vi "Consumer.vi"(8 "error in (no error)":errorcluster, 9 "Data":variant, 10 "Case ID":string, 11 "uService Template in":refnum<class "Detector Manager.lvclass">) -> (0 "error out":errorcluster, 3 "uService Template out":refnum<class "Detector Manager.lvclass">)   [LabVIEW 2026, in "TALOS.lvlib" / "Detector Manager.lvlib" / "Detector Manager.lvclass"]
uses:
  Detector Manager.lvclass
  C:/LabVIEW Code/TALOS/talos/Father of all uServices/Father of all uServices/Father of all uServices.lvclass
  Detector Manager Consumer Case Selector.ctl
  Detector Manager.lvclass/Detector Manager.ctl
  Ancestor/Ancestor/Ancestor.lvclass/Ancestor.ctl
  Father of all uServices/Father of all uServices/Father of all uServices.lvclass/Father of all uServices.ctl
  Father of all uServices/Father of all uServices Messages/Consumer Msg/Consumer Msg.lvclass/Consumer Msg.ctl
  Support VIs/Generate Error.vi
  FGV/Error Memory/Get Error Description.vi
  Support VIs/Get PC name.vi
  Ancestor/Ancestor/Read ID.vi
  Support VIs/Get Class Name.vi
  FGV/Error Memory/Error Memory Core.vi
  <vilib>/AdvancedString/Delimited String to 1D String Array.vi
  <vilib>/AdvancedString/Delimited String to 1D String Array (string).vi
  Support VIs/Circus Root Path.vi
  FGV/Error Memory/Error Crt Lvl checker.vi
  FGV/Error Memory/Error Memory Core.vi/40c8088d-b597-4017-91af-faa98e00292e.vi
  FGV/Error Memory/Error Memory Core.vi/d4a3ab98-063c-4e44-b43d-fbdcfe6c2be2.vi
  Father of all uServices/Father of all uServices/Father of all uServices.lvclass
  C:/LabVIEW Code/TALOS/builds/Actor Framework PPL/Actor Framework.lvlibp/1abvi3w/vi.lib/ActorFramework/Actor/Actor.lvclass
  Support VIs/Global Memory.vi
  <vilib>/Utility/LVClass/Get LV Class Name.vi
  Support VIs/Is in Packed Library.vi
  Support VIs/TALOS Root path.vi
  Support VIs/Read CSV worksheet.vi
  Support VIs/Global Constants.vi
  <vilib>/Utility/error.llb/General Error Handler.vi
  Support VIs/Error Log.vi
  builds/Actor Framework PPL/Actor Framework.lvlibp/1abvi3w/vi.lib/ActorFramework/Actor/Read Self Enqueuer.vi
  <userlib>/_OpenG.lib/lvdata/lvdata.llb/Get Strings from Enum__ogtk.vi
  builds/Actor Framework PPL/Actor Framework.lvlibp/1abvi3w/vi.lib/ActorFramework/Message Enqueuer/Enqueue.vi
  Ancestor/Ancestor/Ancestor.lvclass
  <vilib>/Comparison/Equal/Equal Functor/Equal Functor.lvclass
  Father of all uServices/Father of all uServices Messages/Consumer Msg/Consumer Msg.lvclass
  Classes/Father of all Detectors/Father Of All Detectors.lvclass
  TALOS.lvlib
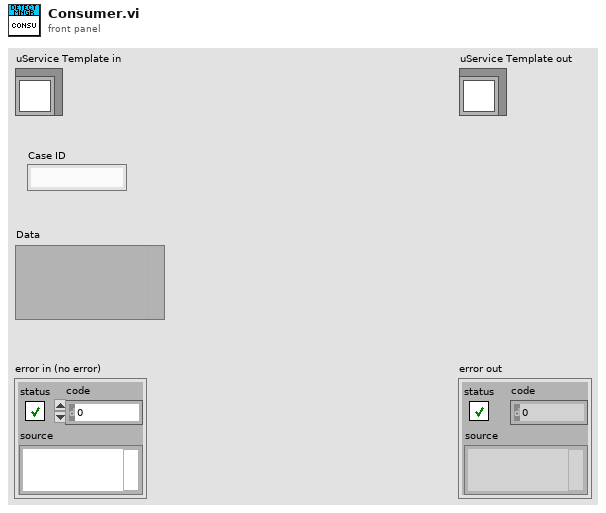
[diagram p1: front panel]
types:
  T1 = typedef "TALOS.lvlib/Detector Manager.lvlib/Detector Manager.lvclass/Detector Manager Consumer Case Selector.ctl" = enum16{"Set Configuration", "Arm", "Acquiring", "Save Data", "Self Check", "Safe Mode", "Init", "Close", "Stop"}
  T2 = typedef "TALOS.lvlib/Father Of All Detectors.lvlib/Father Of All Detectors.lvclass/Detector Settings.ctl" = cluster{"Stop after Save Data?":bool, "Stop before ReArm?":bool}
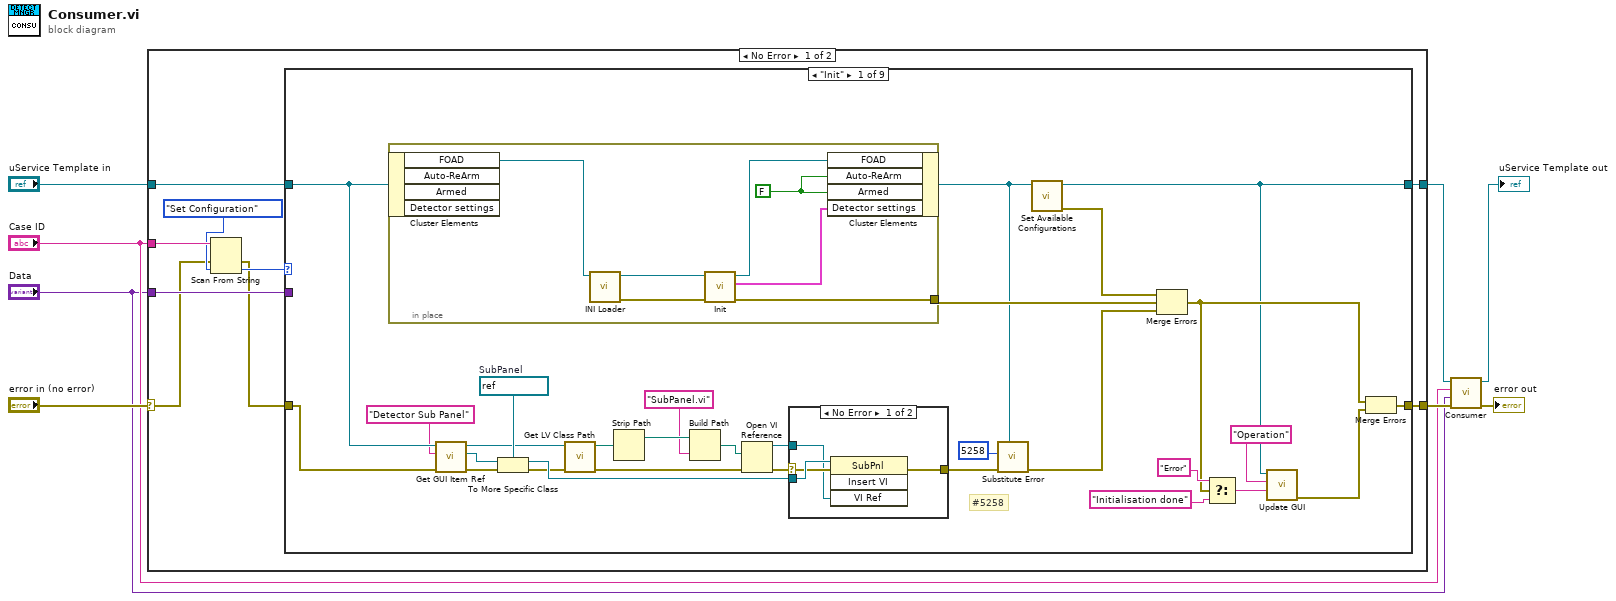
[diagram p0: block diagram]
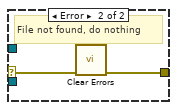
[diagram p2: hidden frame]
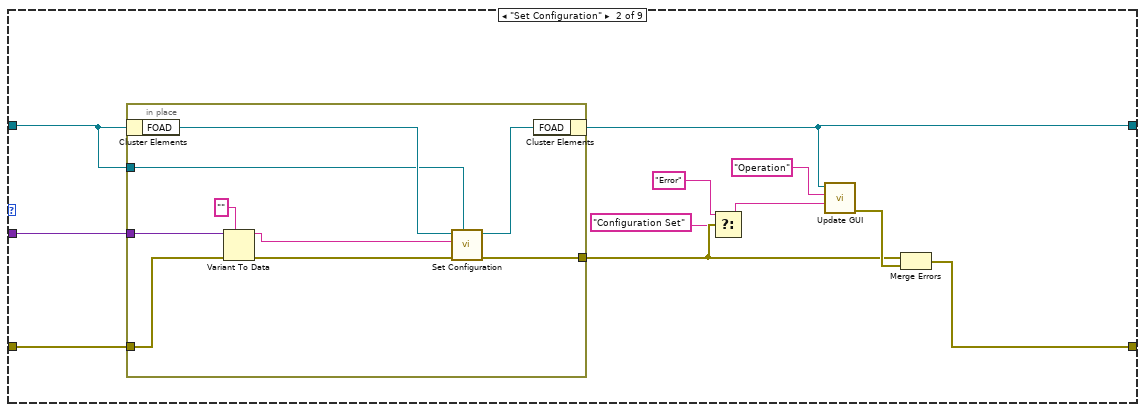
[diagram p3: hidden frame]
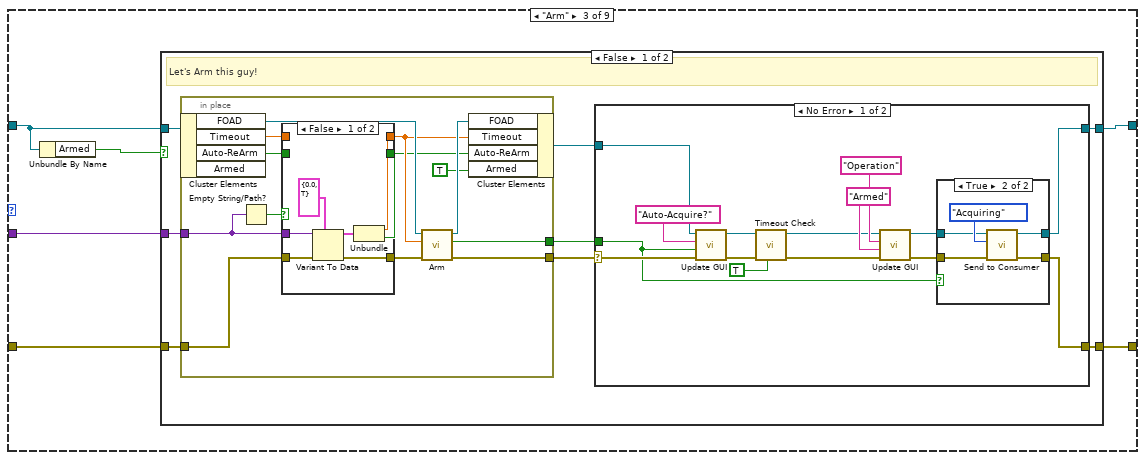
[diagram p4: hidden frame]
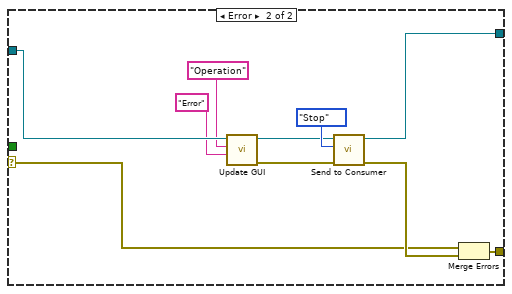
[diagram p7: hidden frame]
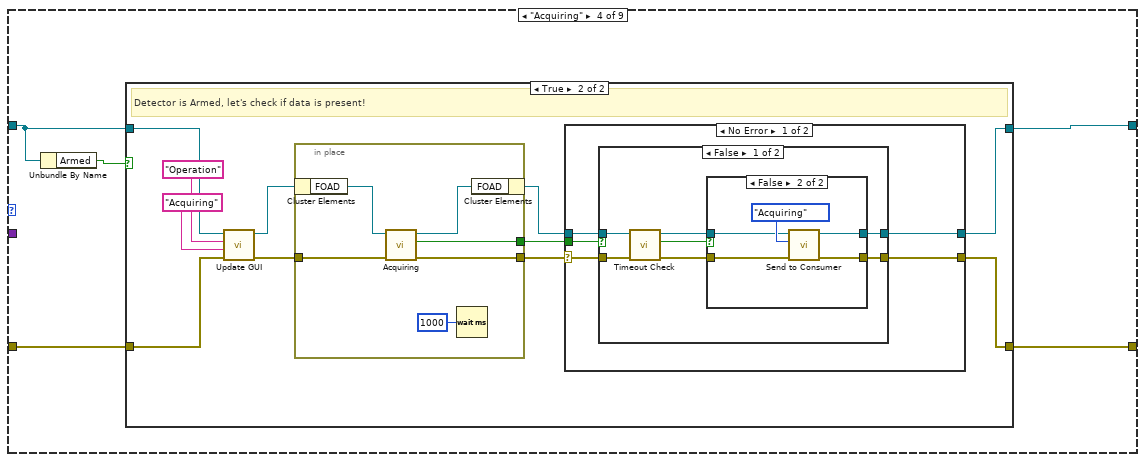
[diagram p9: hidden frame]
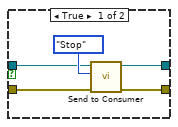
[diagram p11: hidden frame]
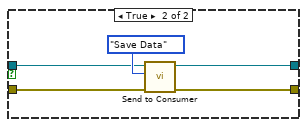
[diagram p12: hidden frame]
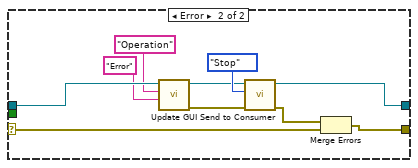
[diagram p13: hidden frame]
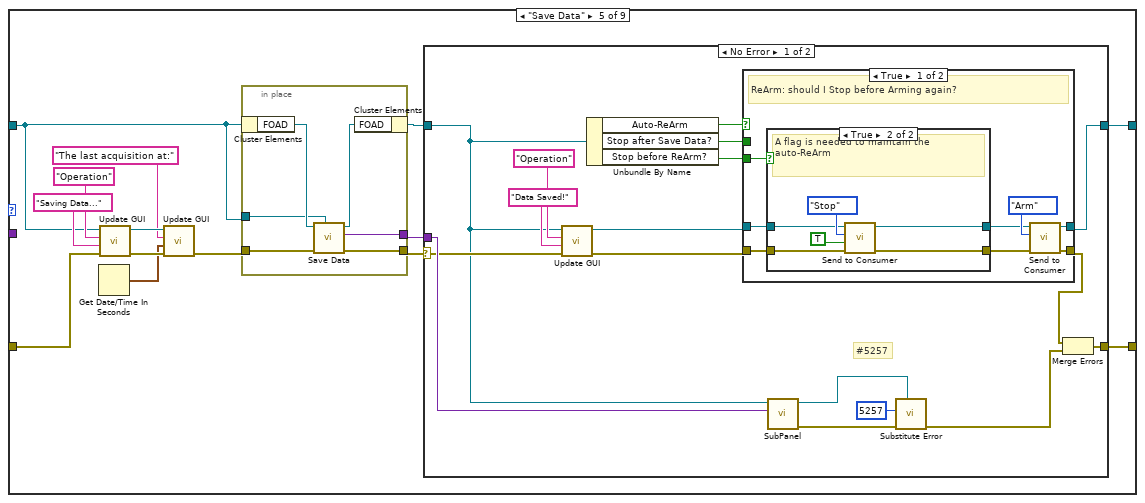
[diagram p14: hidden frame]
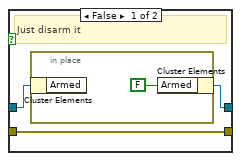
[diagram p15: hidden frame]
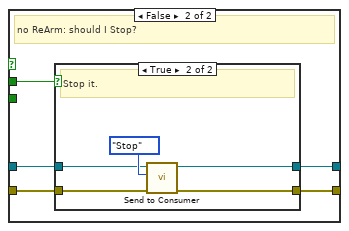
[diagram p16: hidden frame]
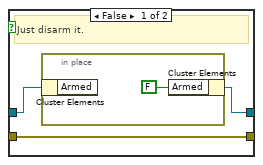
[diagram p17: hidden frame]
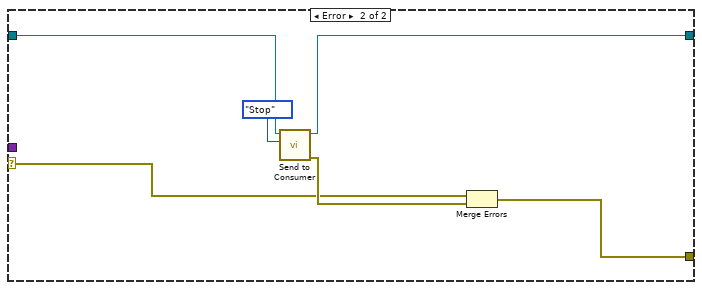
[diagram p18: hidden frame]
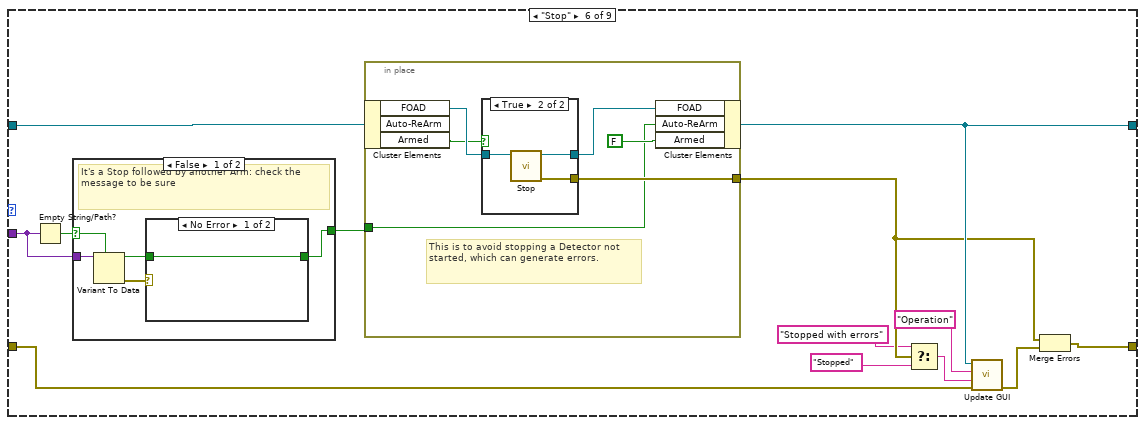
[diagram p19: hidden frame]
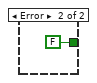
[diagram p20: hidden frame]
diagram:
  n1 = case shown="No Error" "error in (no error)" {
    selector: "error in (no error)" -> [w10 w392]
    tunnel: "uService Template in" -> [w16 w393]
    tunnel: [w14 w393] -> w4
    tunnel: [w15 w392] -> w3
    tunnel: "Case ID" -> [w13 _]
    tunnel: "Data" -> [w17 _]
    frame No Error {
      n2 = Scan From String(input string=w13, error in=w10, default 1=Detector_Manager_Consumer_Case_Selector."Set Configuration") -> (error out=w9:errorcluster, output 1=w11:T1)  [unwired: 2 in, 2 out]
      n3 = case shown="\"Init\"" w11 {
        tunnel: w17 -> [_ w71 w86 _ _ w289 _ w336 w375]
        tunnel: w9 -> [w39 w70 w85 w154 w224 w295 w327 w349 w373]
        tunnel: w16 -> [w40 w61 w82 w153 w218 w300 w328 w350 w374]
        tunnel: [w44 w65 w83 w155 w221 w296 w320 w341 w367] -> w15
        tunnel: [w19 w67 w84 w156 w223 w297 w324 w338 w364] -> w14
        frame "Init" {
          w35 = refnum<vi> refnum  # SubPanel
          # "#5258"
          n4 = in-place "In Place Element Structure" {
            in-place-border: [w59] -> w43
            w58 = FALSE ("Armed")
            n5 = in-place-cluster #1(w40) -> ("FOAD"=w56:refnum<class "Father Of All Detectors.lvclass">)  [unwired: 3 out]
            n6 = call-dynamic "INI Loader.vi"("Father Of All Detectors in"=w56) -> ("error out"=w54:errorcluster, "Father Of All Detectors out"=w55:refnum<class "Father Of All Detectors.lvclass">)  [unwired: 9 in]
            n7 = call-dynamic "Init.vi"("error in (no error)"=w54, "Father Of All Detectors in"=w55) -> ("error out"=w59:errorcluster, "Detector Settings"=w57:T2, "Father Of All Detectors out"=w60:refnum<class "Father Of All Detectors.lvclass">)  [unwired: 7 in]
            n8 = in-place-cluster #1("FOAD"=w60, "Auto-ReArm"=w58, "Armed"=w58, "Detector settings"=w57) -> (w20:refnum<class "Detector Manager.lvclass">)
          }
          n9 = call "Get GUI Item Ref.vi"("error in (no error)"=w39, "FP Item Name"="Detector Sub Panel", "uService Template in"=w40) -> ("error out"=w36:errorcluster, "Ctl Refnum"=w37:refnum<vi>, "uService Template out"=w33:refnum<class "Detector Manager.lvclass">)  [unwired: 6 in]
          n10 = To More Specific Class(target class=w35, reference=w37, error in=w36) -> (specific class reference=w34:refnum<vi>, error out=w32:errorcluster)
          n11 = call <vilib>:"Get LV Class Path.vi"("error in (no error)"=w32, "object"=w33) -> ("error out"=w28:errorcluster, "class path"=w31:path)  [unwired: 8 in]
          n12 = Strip Path(path=w31) -> (stripped path=w30:path)  [unwired: 1 out]
          n13 = Build Path(base path=w30, name or relative path="SubPanel.vi") -> (appended path=w27:path)
          n14 = Open VI Reference(vi path=w27, error in (no error)=w28) -> (vi reference=w25:refnum<vi>, error out=w26:errorcluster)  [unwired: 4 in]
          n15 = case shown="No Error" w26 {
            selector: w26 -> [w50 w53]
            tunnel: w34 -> [w51 _]
            tunnel: w25 -> [w49 _]
            tunnel: [w48 w52] -> w23
            frame No Error {
              n16 = invoke class="SubPnl" method="Insert VI"(reference=w51, error in=w50, "VI Ref"=w49) -> (error out=w48:errorcluster)  [unwired: 1 in, 3 out]
            }
            frame Error {
              # "File not found, do nothing"
              n17 = call <vilib>:"Clear Errors.vi"("error in (no error)"=w53) -> ("error out"=w52:errorcluster)  [unwired: 5 in, 1 out]
            }
          }
          n18 = call "Substitute Error.vi"("LabVIEW Object"=w20, "error in (no error)"=w23, "Error Code"=5258) -> ("error out"=w22:errorcluster)  [unwired: 8 in]
          n19 = call "Set Available Configurations.vi"("Detector Manager in"=w20) -> ("error out"=w18:errorcluster, "Detector Manager out"=w19:refnum<class "Detector Manager.lvclass">)  [unwired: 9 in]
          n20 = Merge Errors(w18, w43, w22) -> (w24:errorcluster)
          n21 = Select(t="Error" ("GUI Item Name"), s=w24, f="Initialisation done" ("GUI Item Name")) -> (s? t:f=w45:string)
          n22 = call "Update GUI.vi"("Data"=w45, "GUI Item Name"="Operation", "uService Template in"=w19) -> ("error out"=w46:errorcluster)  [unwired: 7 in, 1 out]
          n23 = Merge Errors(w24, w46) -> (w44:errorcluster)
        }
        frame "Set Configuration" {
          n24 = in-place "In Place Element Structure" {
            in-place-border: w71 -> [w74]
            in-place-border: w70 -> [w80]
            in-place-border: [w76] -> w64
            in-place-border: w61 -> [w72]
            n25 = in-place-cluster #2(w61) -> ("FOAD"=w79:refnum<class "Father Of All Detectors.lvclass">)
            n26 = Variant To Data(error in=w80, type="", Variant=w74) -> (data=w77:string, error out=w75:errorcluster)
            n27 = call-dynamic "Set Configuration.vi"("Detector Manager"=w72, "error in (no error)"=w75, "Configuration Name"=w77, "Father Of All Detectors in"=w79) -> ("error out"=w76:errorcluster, "Father Of All Detectors out"=w78:refnum<class "Father Of All Detectors.lvclass">)  [unwired: 6 in]
            n28 = in-place-cluster #2("FOAD"=w78) -> (w67:refnum<class "Detector Manager.lvclass">)
          }
          n29 = Select(t="Error" ("f"), s=w64, f="Configuration Set" ("GUI Item Name")) -> (s? t:f=w66:string)
          n30 = call "Update GUI.vi"("Data"=w66, "GUI Item Name"="Operation", "uService Template in"=w67) -> ("error out"=w68:errorcluster)  [unwired: 7 in, 1 out]
          n31 = Merge Errors(w64, w68) -> (w65:errorcluster)
        }
        frame "Arm" {
          n32 = Unbundle By Name(w82) -> ("Armed"=w81:bool)
          n33 = case shown="False" w81 {
            tunnel: w86 -> [w94 _]
            tunnel: w82 -> [w93 w151]
            tunnel: w85 -> [w92 w150]
            tunnel: [w88 w151] -> w84
            tunnel: [w87 w150] -> w83
            frame False {
              # "Let's Arm this guy!"
              n34 = in-place "In Place Element Structure" {
                in-place-border: w94 -> [w101]
                in-place-border: w92 -> [w104]
                in-place-border: [w103] -> w91
                in-place-border: [w102] -> w90
                n35 = in-place-cluster #3(w93) -> ("FOAD"=w107:refnum<class "Father Of All Detectors.lvclass">, "Timeout"=w99:dbl, "Auto-ReArm"=w97:bool)  [unwired: 1 out]
                n36 = Empty String/Path?(string/path=w101) -> (empty?=w100:bool)
                n37 = case shown="False" w100 {
                  tunnel: [w109 w116] -> w98
                  tunnel: [w113 w117] -> w105
                  tunnel: w104 -> [w112 w117]
                  tunnel: w101 -> [w111 _]
                  tunnel: w99 -> [_ w116]
                  tunnel: w97 -> [_ w115]
                  tunnel: [w108 w115] -> w96
                  frame False {
                    n38 = Variant To Data(error in=w112, type=cluster{dbl, bool} {0.0, TRUE}, Variant=w111) -> (data=w114:cluster{dbl, bool}, error out=w113:errorcluster)
                    n39 = Unbundle(w114) -> (w109:dbl, w108:bool)
                  }
                  frame True {
                  }
                }
                n40 = call-dynamic "Arm.vi"("error in (no error)"=w105, "Timeout (s)"=w98, "Father Of All Detectors in"=w107) -> ("error out"=w103:errorcluster, "Acquire?"=w102:bool, "Father Of All Detectors out"=w106:refnum<class "Father Of All Detectors.lvclass">)  [unwired: 6 in]
                n41 = in-place-cluster #3("FOAD"=w106, "Timeout"=w98, "Auto-ReArm"=w96, "Armed"=TRUE) -> (w89:refnum<class "Detector Manager.lvclass">)
              }
              n42 = case shown="No Error" w91 {
                selector: w91 -> [w132 w141]
                tunnel: w90 -> [w130 _]
                tunnel: w89 -> [w129 w149]
                tunnel: [w128 w148] -> w88
                tunnel: [w127 w142] -> w87
                frame No Error {
                  n43 = call "Update GUI.vi"("error in (no error)"=w132, "Data"=w130, "GUI Item Name"="Auto-Acquire?", "uService Template in"=w129) -> ("error out"=w120:errorcluster, "uService Template out"=w122:refnum<class "Detector Manager.lvclass">)  [unwired: 6 in]
                  n44 = call-dynamic "Timeout Check.vi"("Start"=TRUE, "error in (no error)"=w120, "Detector Manager in"=w122) -> ("error out"=w119:errorcluster, "Detector Manager out"=w121:refnum<class "Detector Manager.lvclass">)  [unwired: 6 in, 1 out]
                  n45 = call "Update GUI.vi"("error in (no error)"=w119, "Data"="Armed" ("GUI Item Name"), "GUI Item Name"="Operation", "uService Template in"=w121) -> ("error out"=w125:errorcluster, "uService Template out"=w124:refnum<class "Detector Manager.lvclass">)  [unwired: 6 in]
                  n46 = case shown="True" w130 {
                    tunnel: w125 -> [w133 w138]
                    tunnel: w124 -> [w134 w135]
                    tunnel: [w134 w137] -> w128
                    tunnel: [w133 w136] -> w127
                    frame False {
                    }
                    frame True {
                      n47 = call "Send to Consumer.vi"("error in (no error)"=w138, "Case ID"=Detector_Manager_Consumer_Case_Selector."Acquiring", "uService Template in"=w135) -> ("error out"=w136:errorcluster, "uService Template out"=w137:refnum<class "Detector Manager.lvclass">)  [unwired: 7 in]
                    }
                  }
                }
                frame Error {
                  n48 = call "Update GUI.vi"("Data"="Error" ("GUI Item Name"), "GUI Item Name"="Operation", "uService Template in"=w149) -> ("error out"=w145:errorcluster, "uService Template out"=w140:refnum<class "Detector Manager.lvclass">)  [unwired: 7 in]
                  n49 = call "Send to Consumer.vi"("error in (no error)"=w145, "Case ID"=Detector_Manager_Consumer_Case_Selector."Stop", "uService Template in"=w140) -> ("error out"=w147:errorcluster, "uService Template out"=w148:refnum<class "Detector Manager.lvclass">)  [unwired: 7 in]
                  n50 = Merge Errors(w141, w147) -> (w142:errorcluster)
                }
              }
            }
            frame True {
              # "Armed pressed twice, ignore the second."
            }
          }
        }
        frame "Acquiring" {
          n51 = Unbundle By Name(w153) -> ("Armed"=w152:bool)
          n52 = case shown="True" w152 {
            tunnel: [w158 w169] -> w156
            tunnel: [w157 w168] -> w155
            tunnel: w154 -> [w157 w165]
            tunnel: w153 -> [w158 w159]
            frame False {
              # "This is a spurious message, just ignore it (it can happen if during an acquisition, the Stop button get pressed)."
            }
            frame True {
              # "Detector is Armed, let's check if data is present!"
              n53 = call "Update GUI.vi"("error in (no error)"=w165, "Data"="Acquiring" ("GUI Item Name"), "GUI Item Name"="Operation", "uService Template in"=w159) -> ("error out"=w163:errorcluster, "uService Template out"=w164:refnum<class "Detector Manager.lvclass">)  [unwired: 6 in]
              n54 = in-place "In Place Element Structure" {
                in-place-border: [w210] -> w160
                in-place-border: [w209] -> w162
                in-place-border: w163 -> [w207]
                n55 = in-place-cluster #4(w164) -> ("FOAD"=w212:refnum<class "Father Of All Detectors.lvclass">)
                n56 = call-dynamic "Acquiring.vi"("error in (no error)"=w207, "Father Of All Detectors in"=w212) -> ("error out"=w210:errorcluster, "Ready to Save Data?"=w209:bool, "Father Of All Detectors out"=w211:refnum<class "Father Of All Detectors.lvclass">)  [unwired: 7 in]
                n57 = Wait (ms)(milliseconds to wait=u32 1000) -> ()  [unwired: 1 out]
                n58 = in-place-cluster #4("FOAD"=w211) -> (w161:refnum<class "Detector Manager.lvclass">)
              }
              n59 = case shown="No Error" w160 {
                selector: w160 -> [w170 w200]
                tunnel: [w174 w201] -> w169
                tunnel: [w173 w199] -> w168
                tunnel: w162 -> [w172 _]
                tunnel: w161 -> [w171 w206]
                frame No Error {
                  n60 = case shown="False" w172 {
                    tunnel: [w181 w195] -> w174
                    tunnel: [w180 w194] -> w173
                    tunnel: w171 -> [w179 w192]
                    tunnel: w170 -> [w178 w193]
                    frame False {
                      n61 = call-dynamic "Timeout Check.vi"("error in (no error)"=w178, "Detector Manager in"=w179) -> ("error out"=w177:errorcluster, "Timeout"=w175:bool, "Detector Manager out"=w176:refnum<class "Detector Manager.lvclass">)  [unwired: 7 in]
                      n62 = case shown="False" w175 {
                        tunnel: [w185 w190] -> w181
                        tunnel: [w184 w189] -> w180
                        tunnel: w176 -> [w182 w187]
                        tunnel: w177 -> [w183 w188]
                        frame True {
                          n63 = call "Send to Consumer.vi"("error in (no error)"=w183, "Case ID"=Detector_Manager_Consumer_Case_Selector."Stop", "uService Template in"=w182) -> ("error out"=w184:errorcluster, "uService Template out"=w185:refnum<class "Detector Manager.lvclass">)  [unwired: 7 in]
                        }
                        frame False {
                          n64 = call "Send to Consumer.vi"("error in (no error)"=w188, "Case ID"=Detector_Manager_Consumer_Case_Selector."Acquiring", "uService Template in"=w187) -> ("error out"=w189:errorcluster, "uService Template out"=w190:refnum<class "Detector Manager.lvclass">)  [unwired: 7 in]
                        }
                      }
                    }
                    frame True {
                      n65 = call "Send to Consumer.vi"("error in (no error)"=w193, "Case ID"=Detector_Manager_Consumer_Case_Selector."Save Data", "uService Template in"=w192) -> ("error out"=w194:errorcluster, "uService Template out"=w195:refnum<class "Detector Manager.lvclass">)  [unwired: 7 in]
                    }
                  }
                }
                frame Error {
                  n66 = call "Update GUI.vi"("Data"="Error" ("GUI Item Name"), "GUI Item Name"="Operation", "uService Template in"=w206) -> ("error out"=w202:errorcluster, "uService Template out"=w197:refnum<class "Detector Manager.lvclass">)  [unwired: 7 in]
                  n67 = call "Send to Consumer.vi"("error in (no error)"=w202, "Case ID"=Detector_Manager_Consumer_Case_Selector."Stop", "uService Template in"=w197) -> ("error out"=w198:errorcluster, "uService Template out"=w201:refnum<class "Detector Manager.lvclass">)  [unwired: 7 in]
                  n68 = Merge Errors(w198, w200) -> (w199:errorcluster)
                }
              }
            }
          }
        }
        frame "Save Data" {
          n69 = Get Date/Time In Seconds() -> (seconds since 1Jan1904=w213:timestamp)
          n70 = call "Update GUI.vi"("error in (no error)"=w224, "Data"="Saving Data..." ("GUI Item Name"), "GUI Item Name"="Operation", "uService Template in"=w218) -> ("error out"=w217:errorcluster, "uService Template out"=w216:refnum<class "Detector Manager.lvclass">)  [unwired: 6 in]
          n71 = call "Update GUI.vi"("error in (no error)"=w217, "Data"=w213, "GUI Item Name"="The last acquisition at:", "uService Template in"=w216) -> ("error out"=w214:errorcluster)  [unwired: 6 in, 1 out]
          n72 = in-place "In Place Element Structure" {
            in-place-border: w214 -> [w231]
            in-place-border: [w230] -> w222
            in-place-border: [w229] -> w219
            in-place-border: w218 -> [w227]
            n73 = in-place-cluster #5(w218) -> ("FOAD"=w232:refnum<class "Father Of All Detectors.lvclass">)
            n74 = call-dynamic "Save Data.vi"("Detector Manager"=w227, "error in (no error)"=w231, "Father Of All Detectors in"=w232) -> ("error out"=w229:errorcluster, "Data out"=w230:variant, "Father Of All Detectors out"=w228:refnum<class "Father Of All Detectors.lvclass">)  [unwired: 6 in]
            n75 = in-place-cluster #5("FOAD"=w228) -> (w220:refnum<class "Detector Manager.lvclass">)
          }
          n76 = case shown="No Error" w219 {
            selector: w219 -> [w239 w284]
            tunnel: [w245 w286] -> w223
            tunnel: w222 -> [w244 _]
            tunnel: [w241 w283] -> w221
            tunnel: w220 -> [w238 w282]
            frame No Error {
              # "#5257"
              n77 = call "Update GUI.vi"("error in (no error)"=w239, "Data"="Data Saved!" ("GUI Item Name"), "GUI Item Name"="Operation", "uService Template in"=w238) -> ("error out"=w242:errorcluster, "uService Template out"=w243:refnum<class "Detector Manager.lvclass">)  [unwired: 6 in]
              n78 = Unbundle By Name(w238) -> ("Auto-ReArm"=w247:bool, "Stop after Save Data?"=w237:bool, "Stop before ReArm?"=w236:bool)
              n79 = case shown="True" w247 {
                tunnel: w242 -> [w253 w271]
                tunnel: w243 -> [w254 w272]
                tunnel: [w257 w270] -> w246
                tunnel: [w255 w269] -> w245
                tunnel: w237 -> [_ w268]
                tunnel: w236 -> [w251 _]
                frame True {
                  # "ReArm: should I Stop before Arming again?"
                  n80 = case shown="True" w251 {
                    tunnel: w254 -> [w259 w266]
                    tunnel: [w258 w265] -> w250
                    tunnel: w253 -> [w260 w264]
                    tunnel: [w260 w263] -> w252
                    frame False {
                      # "Just disarm it"
                      n81 = in-place {
                        n82 = in-place-cluster #6(w259) -> ()  [unwired: 1 out]
                        n83 = in-place-cluster #6("Armed"=FALSE) -> (w258:refnum<class "Detector Manager.lvclass">)
                      }
                    }
                    frame True {
                      # "A flag is needed to maintain the auto-ReArm"
                      n84 = call "Send to Consumer.vi"("error in (no error)"=w264, "Data"=TRUE, "Case ID"=Detector_Manager_Consumer_Case_Selector."Stop", "uService Template in"=w266) -> ("error out"=w263:errorcluster, "uService Template out"=w265:refnum<class "Detector Manager.lvclass">)  [unwired: 6 in]
                    }
                  }
                  n85 = call "Send to Consumer.vi"("error in (no error)"=w252, "Case ID"=Detector_Manager_Consumer_Case_Selector."Arm", "uService Template in"=w250) -> ("error out"=w257:errorcluster, "uService Template out"=w255:refnum<class "Detector Manager.lvclass">)  [unwired: 7 in]
                }
                frame False {
                  # "no ReArm: should I Stop?"
                  n86 = case shown="True" w268 {
                    tunnel: w272 -> [w274 w277]
                    tunnel: w271 -> [w275 w281]
                    tunnel: [w275 w280] -> w270
                    tunnel: [w273 w278] -> w269
                    frame False {
                      # "Just disarm it."
                      n87 = in-place {
                        n88 = in-place-cluster #7(w274) -> ()  [unwired: 1 out]
                        n89 = in-place-cluster #7("Armed"=FALSE) -> (w273:refnum<class "Detector Manager.lvclass">)
                      }
                    }
                    frame True {
                      # "Stop it."
                      n90 = call "Send to Consumer.vi"("error in (no error)"=w281, "Case ID"=Detector_Manager_Consumer_Case_Selector."Stop", "uService Template in"=w277) -> ("error out"=w280:errorcluster, "uService Template out"=w278:refnum<class "Detector Manager.lvclass">)  [unwired: 7 in]
                    }
                  }
                }
              }
              n91 = call-dynamic "SubPanel.vi"("Data"=w244, "Detector Manager in"=w238) -> ("error out"=w235:errorcluster, "Detector Manager out"=w234:refnum<class "Detector Manager.lvclass">)  [unwired: 8 in]
              n92 = call "Substitute Error.vi"("LabVIEW Object"=w234, "error in (no error)"=w235, "Error Code"=5257) -> ("error out"=w240:errorcluster)  [unwired: 8 in]
              n93 = Merge Errors(w246, w240) -> (w241:errorcluster)
            }
            frame Error {
              n94 = call "Send to Consumer.vi"("Case ID"=Detector_Manager_Consumer_Case_Selector."Stop", "uService Template in"=w282) -> ("error out"=w285:errorcluster, "uService Template out"=w286:refnum<class "Detector Manager.lvclass">)  [unwired: 8 in]
              n95 = Merge Errors(w284, w285) -> (w283:errorcluster)
            }
          }
        }
        frame "Stop" {
          n96 = Empty String/Path?(string/path=w289) -> (empty?=w290:bool)
          n97 = case shown="False" w290 {
            selector: w290 -> [w304 _]
            tunnel: w289 -> [w305 _]
            tunnel: [w301 FALSE] -> w288
            frame False {
              # "It's a Stop followed by another Arm: check the message to be sure"
              n98 = Variant To Data(type=w304, Variant=w305) -> (data=w302:bool, error out=w303:errorcluster)  [unwired: 1 in]
              n99 = case shown="No Error" w303 {
                tunnel: w302 -> [w306 _]
                tunnel: [w306 FALSE] -> w301
                frame No Error {
                }
                frame Error {
                }
              }
            }
            frame True {
              # "This is a real Stop, put Auto-ReArm to False"
            }
          }
          n100 = in-place "In Place Element Structure" {
            in-place-border: [w312] -> w294
            in-place-border: w288 -> [w309]
            # "This is to avoid stopping a Detector not started, which can generate errors."
            n101 = in-place-cluster #8(w300) -> ("FOAD"=w314:refnum<class "Father Of All Detectors.lvclass">, "Armed"=w310:bool)  [unwired: 1 out]
            n102 = case shown="True" w310 {
              tunnel: w314 -> [w316 w319]
              tunnel: [w316 w318] -> w313
              tunnel: [errorcluster {"status"=FALSE, "code"=0, "source"=""} ("error out") w317] -> w312
              frame False {
              }
              frame True {
                n103 = call-dynamic "Stop.vi"("Father Of All Detectors in"=w319) -> ("error out"=w317:errorcluster, "Father Of All Detectors out"=w318:refnum<class "Father Of All Detectors.lvclass">)  [unwired: 9 in]
              }
            }
            n104 = in-place-cluster #8("FOAD"=w313, "Auto-ReArm"=w309, "Armed"=FALSE) -> (w297:refnum<class "Detector Manager.lvclass">)
          }
          n105 = Select(t="Stopped with errors", s=w294, f="Stopped" ("GUI Item Name")) -> (s? t:f=w291:string)
          n106 = call "Update GUI.vi"("error in (no error)"=w295, "Data"=w291, "GUI Item Name"="Operation", "uService Template in"=w297) -> ("error out"=w298:errorcluster)  [unwired: 6 in, 1 out]
          n107 = Merge Errors(w294, w298) -> (w296:errorcluster)
        }
        frame "Close" {
          n108 = in-place "In Place Element Structure" {
            in-place-border: w327 -> [w332]
            in-place-border: [w331] -> w329
            w330 = FALSE ("Armed")
            n109 = in-place-cluster #9(w328) -> ("FOAD"=w334:refnum<class "Father Of All Detectors.lvclass">)  [unwired: 2 out]
            n110 = call-dynamic "Close.vi"("error in (no error)"=w332, "Father Of All Detectors in"=w334) -> ("error out"=w331:errorcluster, "Father Of All Detectors out"=w333:refnum<class "Father Of All Detectors.lvclass">)  [unwired: 8 in]
            n111 = in-place-cluster #9("FOAD"=w333, "Auto-ReArm"=w330, "Armed"=w330) -> (w324:refnum<class "Detector Manager.lvclass">)
          }
          n112 = Select(t="Error", s=w329, f="Closed" ("GUI Item Name")) -> (s? t:f=w323:string)
          n113 = call "Update GUI.vi"("Data"=w323, "GUI Item Name"="Operation", "uService Template in"=w324) -> ("error out"=w325:errorcluster)  [unwired: 7 in, 1 out]
          n114 = Merge Errors(w329, w325) -> (w320:errorcluster)
        }
        frame "Self Check" {
          # "If the variant is empty, it means it is used to manually perform the check with the button. It's a different case than the EH Ready to Launch because it does not restitute the Go-NoGo."
          n115 = in-place "In Place Element Structure" {
            in-place-border: w349 -> [w361]
            in-place-border: [w360] -> w343
            in-place-border: [w359] -> w337
            n116 = in-place-cluster #10(w350) -> ("FOAD"=w363:refnum<class "Father Of All Detectors.lvclass">)
            n117 = call-dynamic "Self Check.vi"("error in (no error)"=w361, "Father Of All Detectors in"=w363) -> ("error out"=w360:errorcluster, "OK?"=w359:bool, "Father Of All Detectors out"=w362:refnum<class "Father Of All Detectors.lvclass">)  [unwired: 7 in]
            n118 = in-place-cluster #10("FOAD"=w362) -> (w339:refnum<class "Detector Manager.lvclass">)
          }
          n119 = Select(t="Self Check Passed!" ("GUI Item Name"), s=w337, f="Self Check NOT Passed!" ("GUI Item Name")) -> (s? t:f=w347:string)
          n120 = call "Update GUI.vi"("Data"=w347, "GUI Item Name"="Operation", "uService Template in"=w339) -> ("error out"=w346:errorcluster, "uService Template out"=w340:refnum<class "Detector Manager.lvclass">)  [unwired: 7 in]
          n121 = Merge Errors(w343, w346) -> (w342:errorcluster)
          n122 = Empty String/Path?(string/path=w336) -> (empty?=w335:bool)
          n123 = case shown="False" w335 {
            tunnel: w342 -> [w356 w357]
            tunnel: [w355 w357] -> w341
            tunnel: w340 -> [w354 w358]
            tunnel: [w353 w358] -> w338
            tunnel: w337 -> [w352 _]
            tunnel: w336 -> [w351 _]
            frame False {
              n124 = call-dynamic "Go-NoGo.vi"("error in (no error)"=w356, "Go-NoGo Data"=w351, "Go?"=w352, "Father of all uServices in"=w354) -> ("error out"=w355:errorcluster, "Father of all uServices out"=w353:refnum<class "Detector Manager.lvclass">)  [unwired: 6 in]
            }
            frame True {
            }
          }
        }
        frame "Safe Mode" {
          n125 = in-place "In Place Element Structure" {
            in-place-border: w375 -> [_]
            in-place-border: w373 -> [w384]
            in-place-border: [w376] -> w366
            w383 = FALSE ("Auto-ReArm")
            # "This is to avoid stopping a Detector not started, which can generate errors."
            n126 = in-place-cluster #11(w374) -> ("FOAD"=w385:refnum<class "Father Of All Detectors.lvclass">, "Armed"=w382:bool)  [unwired: 1 out]
            n127 = call-dynamic "Safe Mode.vi"("error in (no error)"=w384, "Father Of All Detectors in"=w385) -> ("error out"=w377:errorcluster, "Stop?"=w380:bool, "Father Of All Detectors out"=w379:refnum<class "Father Of All Detectors.lvclass">)  [unwired: 7 in]
            n128 = And(x=w382, y=w380) -> (x .and. y?=w381:bool)
            n129 = case shown="True" w381 {
              tunnel: w379 -> [w387 w391]
              tunnel: [w387 w390] -> w378
              tunnel: [w386 w389] -> w376
              tunnel: w377 -> [w386 w388]
              frame False {
              }
              frame True {
                n130 = call-dynamic "Stop.vi"("error in (no error)"=w388, "Father Of All Detectors in"=w391) -> ("error out"=w389:errorcluster, "Father Of All Detectors out"=w390:refnum<class "Father Of All Detectors.lvclass">)  [unwired: 8 in]
              }
            }
            n131 = in-place-cluster #11("FOAD"=w378, "Auto-ReArm"=w383, "Armed"=w383) -> (w365:refnum<class "Detector Manager.lvclass">)
          }
          n132 = Select(t="ERROR IN ENABLING SAFE MODE" ("GUI Item Name"), s=w366, f="SAFE MODE ENABLED" ("GUI Item Name")) -> (s? t:f=w368:string)
          n133 = call "Update GUI.vi"("Data"=w368, "GUI Item Name"="Operation", "uService Template in"=w365) -> ("error out"=w371:errorcluster, "uService Template out"=w364:refnum<class "Detector Manager.lvclass">)  [unwired: 7 in]
          n134 = Merge Errors(w366, w371) -> (w367:errorcluster)
        }
      }
    }
    frame Error {
    }
  }
  n135 = call-parent "Consumer.vi"("error in (no error)"=w3, "Data"="Data", "Case ID"="Case ID", "uService Template in"=w4) -> ("error out"=→"error out":errorcluster, "uService Template out"=→"uService Template out":refnum<class "Detector Manager.lvclass">)  [unwired: 6 in]
